vi "Configure Monitor.vi"(8 "error in (no error)":errorcluster, 9 "Parameter (0: OFF)":i32(ring) items=["OFF", "Z", "D", "Q", "THR", "THD", "R", "X", "G", "B", "Y", "ABS", "PER", "VAC", "IAC"], 10 "Monitor (1)":i32(ring)=1 items=["1"=1, "2"=2], 11 "VISA resource name":refnum<visa-resource-name>) -> (0 "error out":errorcluster, 3 "VISA resource name out":refnum<visa-resource-name>)   [LabVIEW 2021, in "LCR Meter.lvlib"]
doc: "Sets the monitor1 and monitor2 parameter."
uses:
  LCR Meter.lvlib
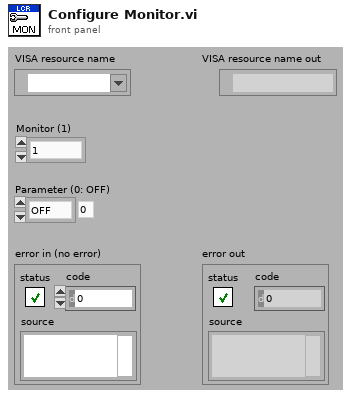
[diagram p1: front panel]
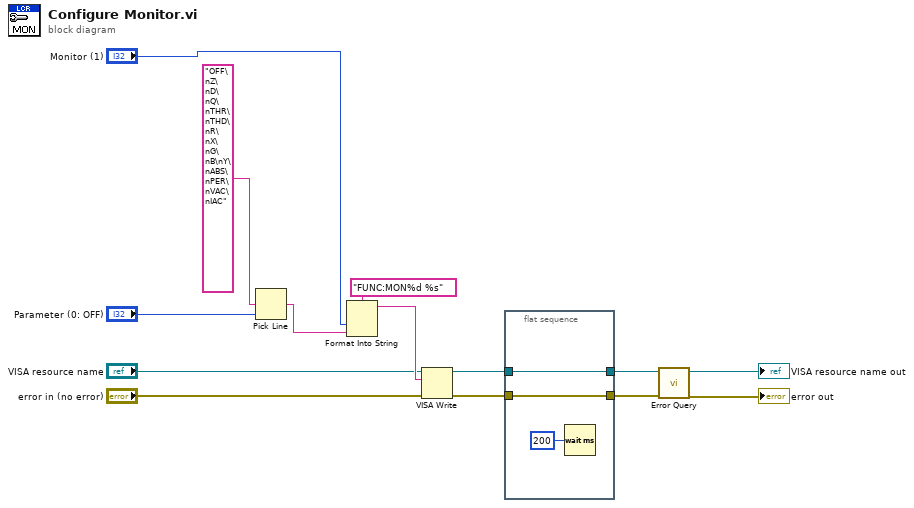
[diagram p0: block diagram]
diagram:
  n1 = Pick Line(multi-line string="OFF\nZ\nD\nQ\nTHR\nTHD\nR\nX\nG\nB\nY\nABS\nPER\nVAC\nIAC", line index="Parameter (0: OFF)") -> (output string=w10:string)  [unwired: 1 in]
  n2 = Format Into String(format string="FUNC:MON%d %s", "Monitor (1)", w10) -> (resulting string=w9:string)  [unwired: 2 in, 1 out]
  n3 = VISA Write(VISA resource name="VISA resource name", write buffer=w9, error in (no error)="error in (no error)") -> (VISA resource name out=w4:refnum<visa-resource-name>, error out=w2:errorcluster)  [unwired: 1 out]
  n4 = flat-sequence {
    tunnel: w4 -> [w17]
    tunnel: [w17] -> w3
    tunnel: w2 -> [w16]
    tunnel: [w16] -> w1
    frame #0 {
      n5 = Wait (ms)(milliseconds to wait=u32 200) -> ()  [unwired: 1 out]
    }
  }
  n6 = call "Error Query.vi"("error in (no error)"=w1, "VISA resource name"=w3) -> ("error out"=→"error out":errorcluster, "VISA resource name out"=→"VISA resource name out":refnum<visa-resource-name>)  [unwired: 6 in, 2 out]
